vi "Functional Post Analysis.vi"(0 "Saving Path":path, 1 "Sensors":T2(array[cluster])=[{"Sensor Name"="", "Sensor Info"={"Manufacturer"="", "Model"="", "Serial Number"=""}, "Last Cal Info"={"Last Calibration Date"=0.0, "Calibrator"="", "Cal Duration"=0}, "Voltage Range"={"High Limit"=0.0, "Low Limit"=0.0}, "EGU Range"={"High Limit"=0.0, "Low Limit"=0.0}, "Units"="Volts", "Calibration Type"=enum."Calibrate Analog", "EGU List"=[], "Voltage List"=[], "Coefficients"=[], "Order"=0, "Algorithm"=enum."SVD", "Max Error % of Full Scale"=0.0, "Max Mean Squared Error"=0.0, "Use Error %"=FALSE, "Use MSE"=FALSE, "Allow Manual Entry"=FALSE, "Max Stability Error"=0.0, "Max Error % of Reading"=0.0, "Use Error % of Reading"=FALSE}], 2 "Config":T3={"DAQ Settings"={"Trigger Type"=enum."Manual", "Trigger Samples"=0, "Pretrigger Samples"=0, "Trigger Interval"=0.0, "Time Units"=FALSE, "Auto Save"=FALSE, "Sample Rate"=7.0, "Select Analog"=FALSE, "Trigger Value"=0.0, "Trigger Stop Method"=enum."Use Samples Value to Stop Trigger", "Rate Sec/Min"=FALSE, "Save Mode"=enum."Single File", "File Size Limit"=0.0, "Log File Type"=enum."Basic", "Trigger Data Index"=0}, "Channels"=[{"Channel"="", "Type"="", "Acquire"=FALSE, "Name"="", "Sensor"="", "Data Index"=0}, {"Channel"="", "Type"="", "Acquire"=FALSE, "Name"="", "Sensor"="", "Data Index"=0}, {"Channel"="", "Type"="", "Acquire"=FALSE, "Name"="", "Sensor"="", "Data Index"=0}, {"Channel"="", "Type"="", "Acquire"=FALSE, "Name"="", "Sensor"="", "Data Index"=0}], "Header"={"TA Number"="", "Test Name"="", "Serial Number"="", "Technician"=""}, "Graph Settings"={"Graph Labels"=[], [], [], [], [], [], [], [], [], [], [], [], [], "Graph Toggles"=[], "Axis Toggles"=[], "Graph Range"=enum."1"}, "Test Limits"=[{"Channel Acquired?"=TRUE, "RMS?"=FALSE, "Pk-Pk"=FALSE, "Frequency"=TRUE, "EU High Limit 1"=0.0, "EU Low Limit 1"=0.0, "EU High Limit 2"=0.0, "EU Low Limit 2"=0.0, "RMS High Limit"=0.0, "RMS Low Limit"=0.0, "Pk-Pk High Limit "=0.0, "Pk-Pk Low Limit"=0.0, "Frequency High Limit"=1.0, "Frequency Low Limit"=0.0}, {"Channel Acquired?"=TRUE, "RMS?"=FALSE, "Pk-Pk"=FALSE, "Frequency"=FALSE, "EU High Limit 1"=1.0, "EU Low Limit 1"=0.0, "EU High Limit 2"=0.0, "EU Low Limit 2"=0.0, "RMS High Limit"=0.0, "RMS Low Limit"=0.0, "Pk-Pk High Limit "=0.0, "Pk-Pk Low Limit"=0.0, "Frequency High Limit"=0.0, "Frequency Low Limit"=0.0}, {"Channel Acquired?"=TRUE, "RMS?"=FALSE, "Pk-Pk"=FALSE, "Frequency"=TRUE, "EU High Limit 1"=0.0, "EU Low Limit 1"=0.0, "EU High Limit 2"=0.0, "EU Low Limit 2"=0.0, "RMS High Limit"=0.0, "RMS Low Limit"=0.0, "Pk-Pk High Limit "=0.0, "Pk-Pk Low Limit"=0.0, "Frequency High Limit"=1.0, "Frequency Low Limit"=0.0}, {"Channel Acquired?"=TRUE, "RMS?"=FALSE, "Pk-Pk"=FALSE, "Frequency"=FALSE, "EU High Limit 1"=1.0, "EU Low Limit 1"=0.0, "EU High Limit 2"=0.0, "EU Low Limit 2"=0.0, "RMS High Limit"=0.0, "RMS Low Limit"=0.0, "Pk-Pk High Limit "=0.0, "Pk-Pk Low Limit"=0.0, "Frequency High Limit"=0.0, "Frequency Low Limit"=0.0}], "All Type Info"=[{"Type Name"="Type Name", "Type Signal Names"=["Signal 1", "Signal 2"], "# Signals"=2, "# Parts"=2, "Part Info"=[{"Part Number"="Part 1", "Channel Indexes"=[0, 1], "Enabled?"=TRUE}, {"Part Number"="Part 2", "Channel Indexes"=[2, 3], "Enabled?"=TRUE}]}], "Save Mode"=enum."Single File"} {"DAQ Settings"."Trigger Interval" min=0.0; "DAQ Settings"."Pretrigger Samples" min=0; "DAQ Settings"."Trigger Samples" min=0}, 3 "Frequency Coefficients":cluster{"Coefficients":dbl[]}[](array[cluster]), 7 "Functional Test Data":T1) -> (4 "Array":string[][](array[string]))   [LabVIEW 2019]
uses:
  <vilib>/Utility/file.llb/Read From Spreadsheet File (string).vi
  Type Defs and Controls/Trigger Stop Method.ctl
  Type Defs and Controls/DAQ Settings.ctl
  Type Defs and Controls/Header.ctl
  Type Defs and Controls/Channel Config.ctl
  Type Defs and Controls/Graph Settings Type Def.ctl
  Type Defs and Controls/Test Limits.ctl
  Type Defs and Controls/Sensor Config.ctl
  Type Defs and Controls/Part Info.ctl
  Type Defs and Controls/All Part Info.ctl
  Type Defs and Controls/Functional Info.ctl
  Type Defs and Controls/Log File Type.ctl
panel:
  out "number":sgl[][](array[numeric])
  out "error out":errorcluster
  # "EGU"
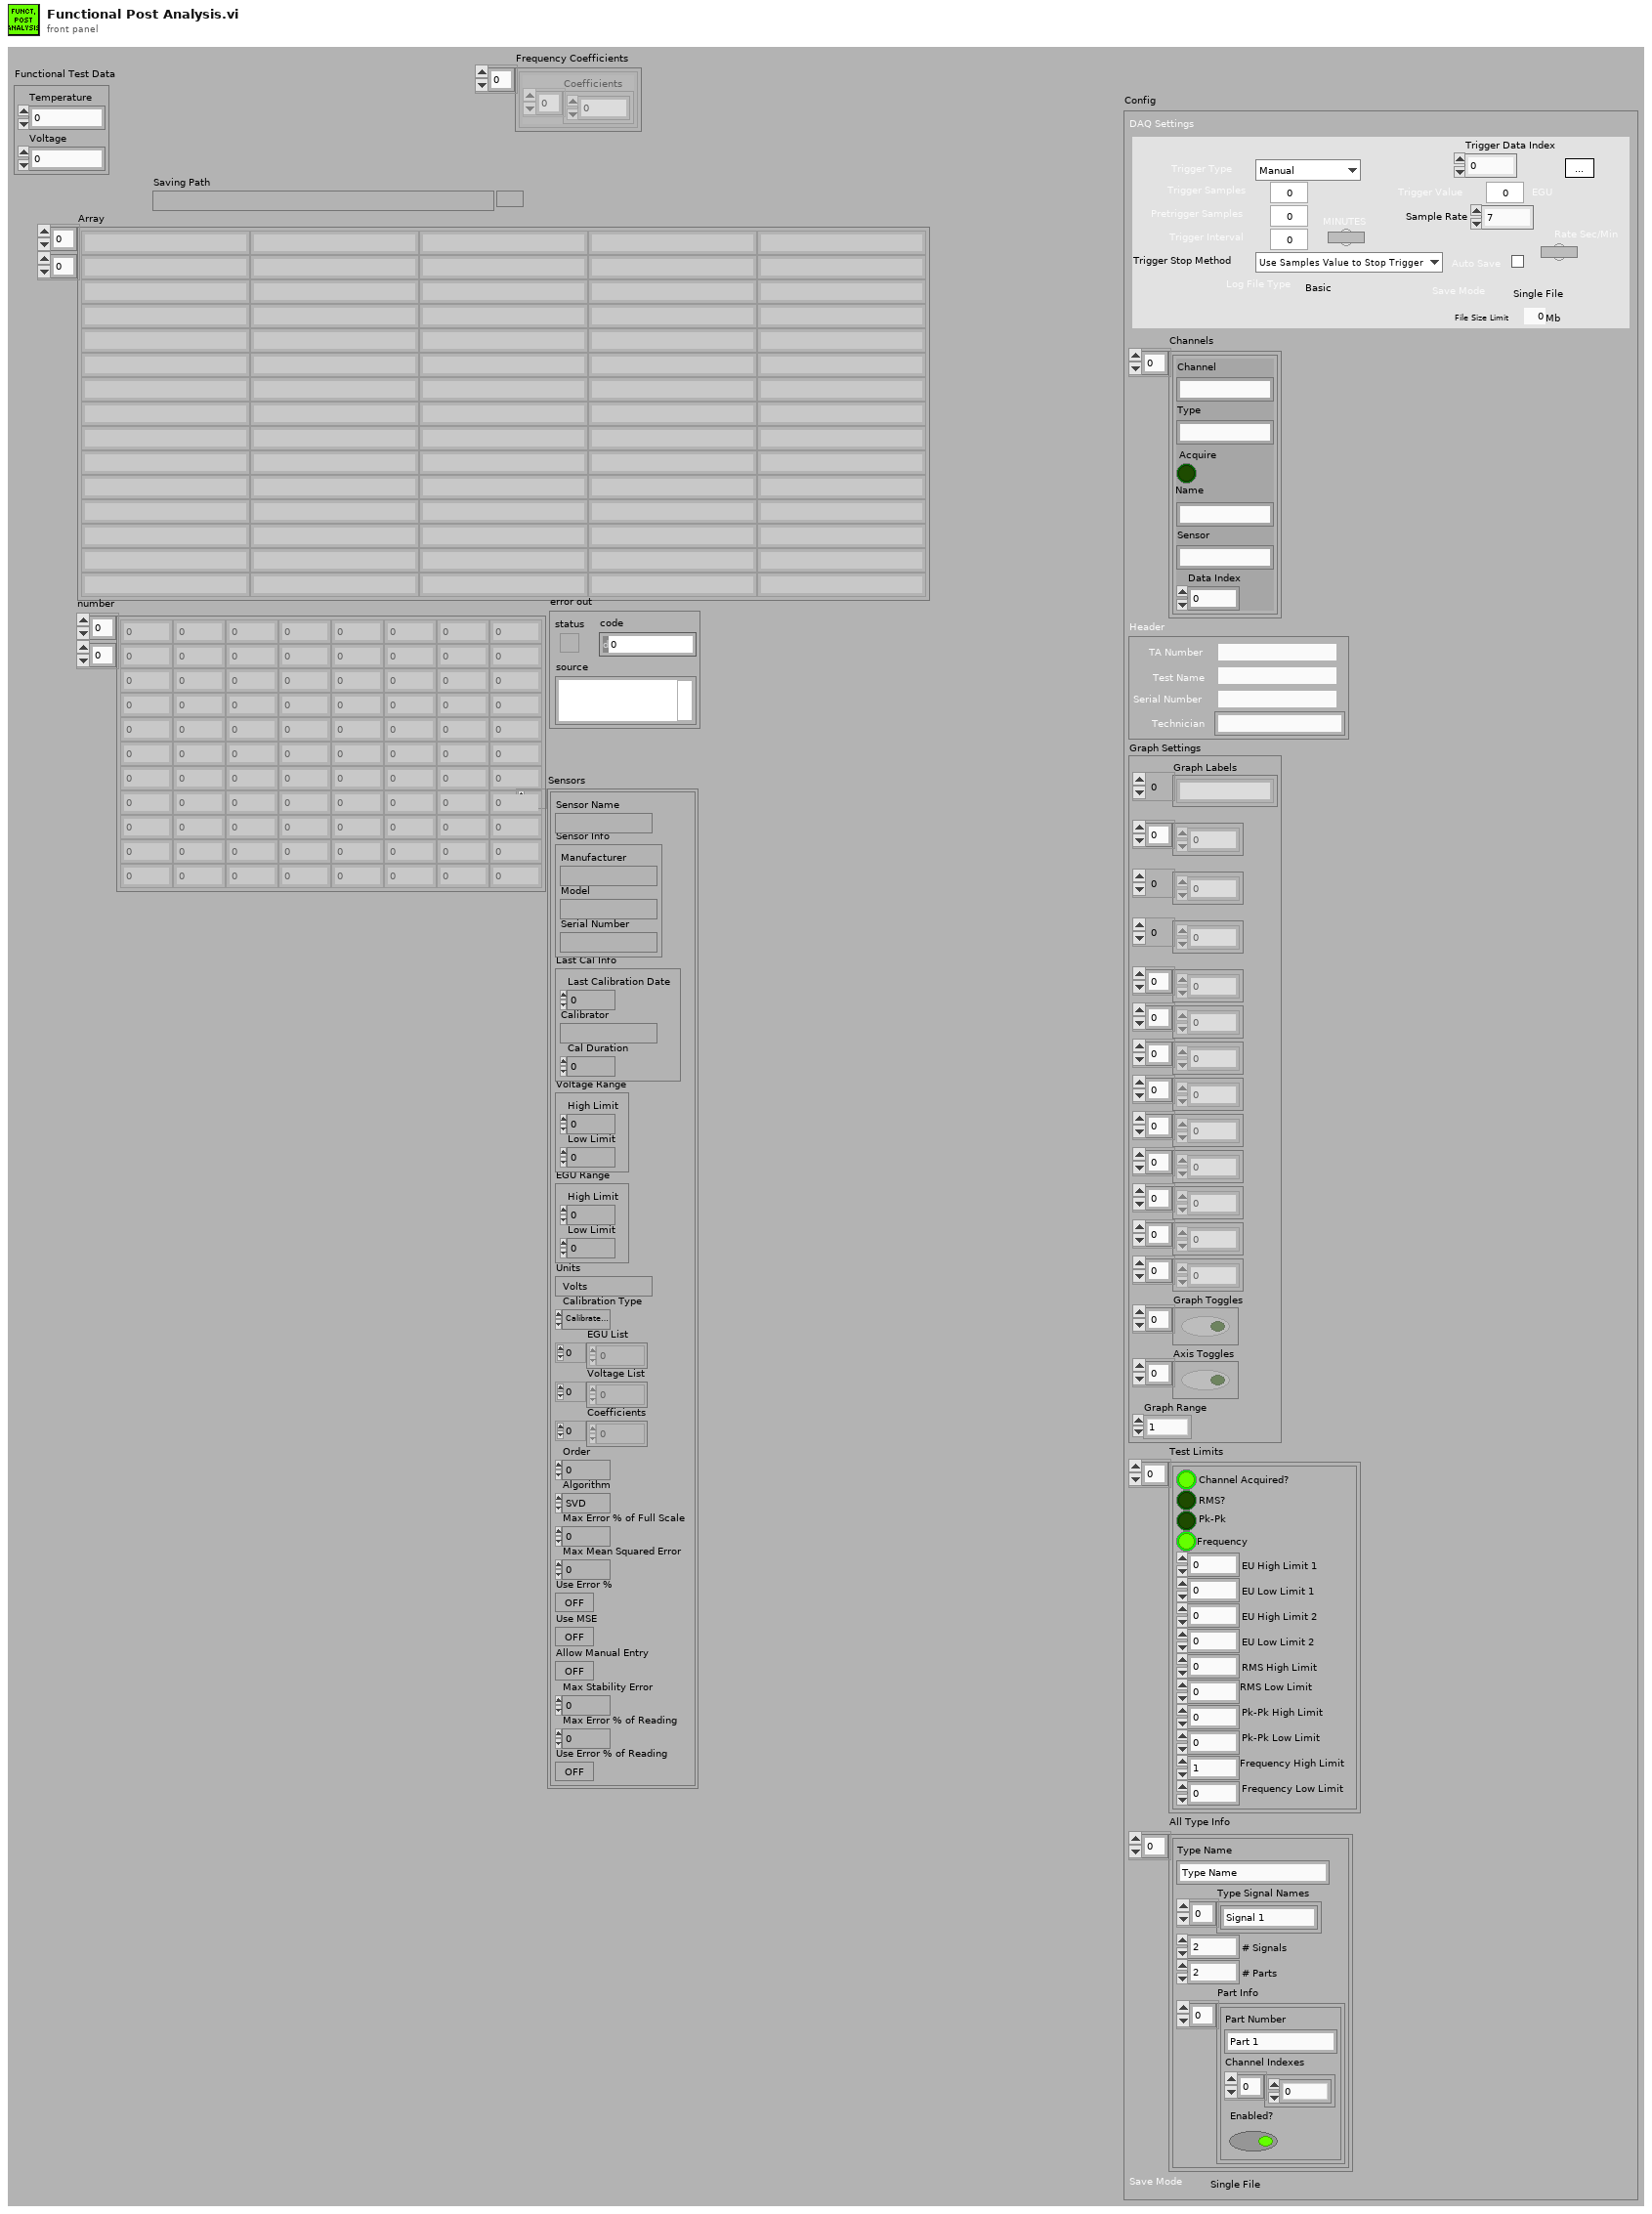
[diagram p1: front panel]
types:
  T1 = typedef "Functional Info.ctl" = cluster{"Temperature":dbl, "Voltage":dbl}
  T2 = cluster{"Sensor Name":string, "Sensor Info":cluster{"Manufacturer":string, "Model":string, "Serial Number":string}, "Last Cal Info":cluster{"Last Calibration Date":dbl, "Calibrator":string, "Cal Duration":i32}, "Voltage Range":cluster{"High Limit":dbl, "Low Limit":dbl}, "EGU Range":cluster{"High Limit":dbl, "Low Limit":dbl}, "Units":string, "Calibration Type":enum16{"Calibrate Analog", "Compare Analog Calibration"}, "EGU List":dbl[], "Voltage List":dbl[], "Coefficients":dbl[], "Order":i32, "Algorithm":enum32{"SVD", "Givens", "Givens2", "Householder", "LU Decomposition", "Cholesky"}, "Max Error % of Full Scale":dbl, "Max Mean Squared Error":dbl, "Use Error %":bool, "Use MSE":bool, "Allow Manual Entry":bool, "Max Stability Error":dbl, "Max Error % of Reading":dbl, "Use Error % of Reading":bool}[]
  T3 = typedef "Sensor Config.ctl" = cluster{"DAQ Settings":T4, "Channels":T7[], "Header":T8, "Graph Settings":T9, "Test Limits":T10[], "All Type Info":T11, "Save Mode":enum16{"Single File", "Segmented Files", "New File at Midnight"}}
  T4 = typedef "DAQ Settings.ctl" = cluster{"Trigger Type":enum16{"Manual", "Timed", "Analog Rising", "Analog Falling"}, "Trigger Samples":i32, "Pretrigger Samples":i32, "Trigger Interval":dbl, "Time Units":bool, "Auto Save":bool, "Sample Rate":dbl, "Select Analog":bool, "Trigger Value":dbl, "Trigger Stop Method":T5, "Rate Sec/Min":bool, "Save Mode":enum16{"Single File", "Segmented Files", "New File at Midnight"}, "File Size Limit":dbl, "Log File Type":T6, "Trigger Data Index":u32}
  T5 = typedef "Trigger Stop Method.ctl" = enum16{"Use Samples Value to Stop Trigger", "Use Threshold to Stop Trigger"}
  T6 = typedef "Log File Type.ctl" = enum16{"Basic", "RTS"}
  T7 = typedef "Channel Config.ctl" = cluster{"Channel":string, "Type":string, "Acquire":bool, "Name":string, "Sensor":string, "Data Index":u32}
  T8 = typedef "Header.ctl" = cluster{"TA Number":string, "Test Name":string, "Serial Number":string, "Technician":string}
  T9 = typedef "Graph Settings Type Def.ctl" = cluster{"Graph Labels":string[], u8[], i16[], u32[], u8[], u8[], u8[], u32[], u8[], u8[], u8[], dbl[], dbl[], "Graph Toggles":bool[], "Axis Toggles":bool[], "Graph Range":enum16{"1", "2", "3", "4", "5", "10", "15", "30", "60"}}
  T10 = typedef "Test Limits.ctl" = cluster{"Channel Acquired?":bool, "RMS?":bool, "Pk-Pk":bool, "Frequency":bool, "EU High Limit 1":dbl, "EU Low Limit 1":dbl, "EU High Limit 2":dbl, "EU Low Limit 2":dbl, "RMS High Limit":dbl, "RMS Low Limit":dbl, "Pk-Pk High Limit ":dbl, "Pk-Pk Low Limit":dbl, "Frequency High Limit":dbl, "Frequency Low Limit":dbl}
  T11 = typedef "All Part Info.ctl" = cluster{"Type Name":string, "Type Signal Names":string[], "# Signals":i32, "# Parts":i32, "Part Info":T12[]}[]
  T12 = typedef "Part Info.ctl" = cluster{"Part Number":string, "Channel Indexes":u16[], "Enabled?":bool}
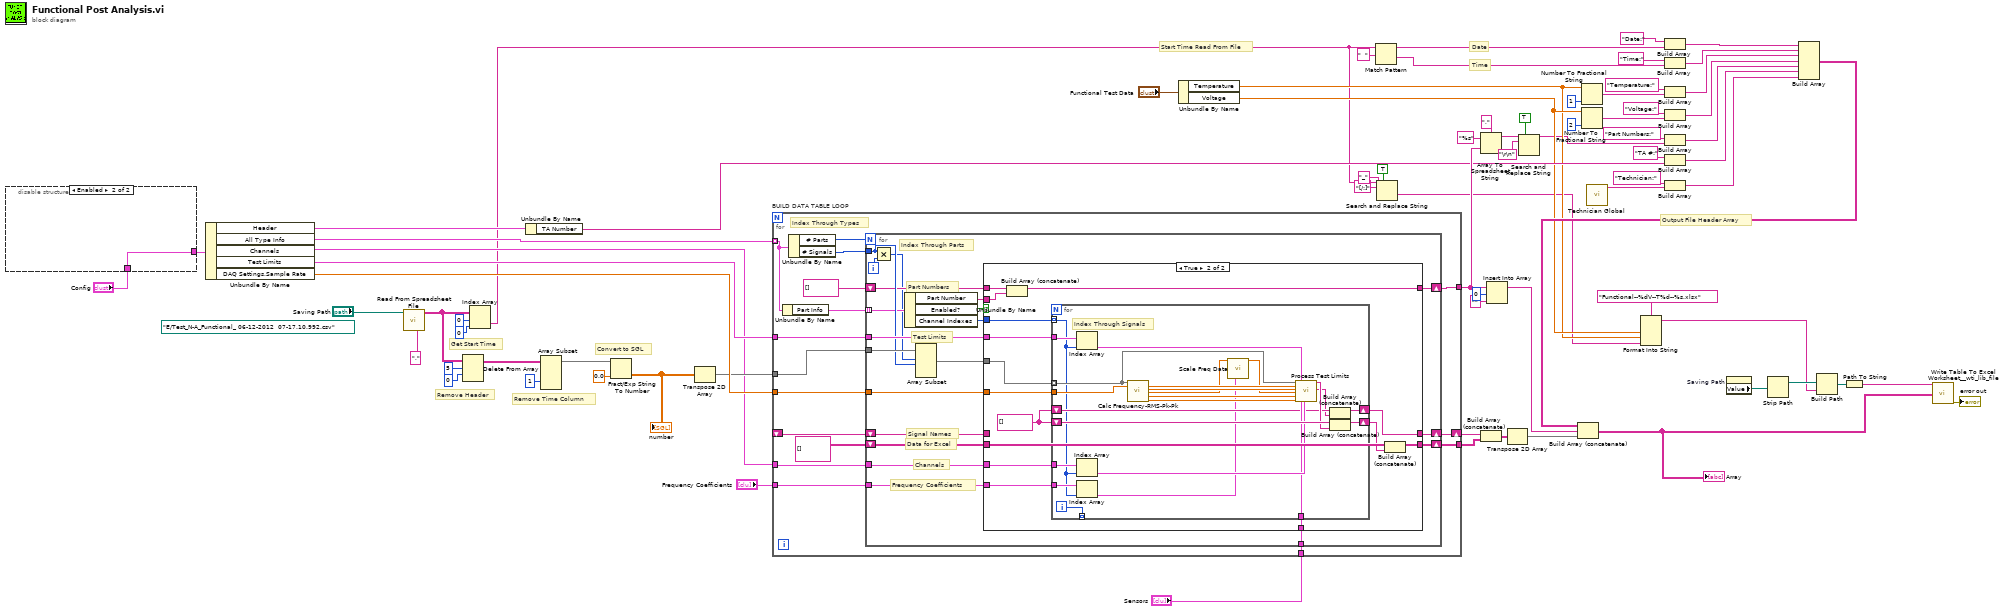
[diagram p0: block diagram]
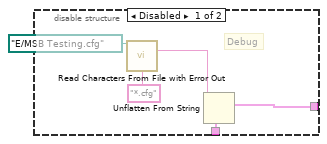
[diagram p2: hidden frame]
diagram:
  (unwired) path "E:/Test_N-A_Functional_ 06-12-2012  07-17.10.992.csv" ("file path (dialog if empty)")
  # "Start Time Read From File"
  # "Time"
  # "Date"
  # "Output File Header Array"
  # "Get Start Time"
  # "Remove Header"
  # "Convert to SGL"
  # "Remove Time Column"
  n1 = disable-structure shown="Enabled" {
    disable-tunnel: "Config" -> [w79 w82]
    disable-tunnel: [w78 w82] -> w2
    frame Disabled {
      # "Debug"
      n2 = call "Read Characters From File with Error Out.vi"("file path (dialog if empty)"=path "E:/MSB Testing.cfg", "[pattern]"="*.cfg") -> ("character string"=w80:string)  [unwired: 9 in, 4 out]
      n3 = Unflatten From String(type=w79, binary string=w80) -> (value=w78:T3)  [unwired: 3 in, 2 out]
    }
    frame Enabled {
    }
  }
  n4 = Unbundle By Name(w2) -> ("Header"=w57:T8, "All Type Info"=w68:T11, "Channels"=w66:T7[], "Test Limits"=w67:T10[], "DAQ Settings.Sample Rate"=w70:dbl)
  n5 = call-poly <vilib>:"Read From Spreadsheet File.vi"("delimiter (\\t)"="," ("delimiter (\\t)"), "file path (dialog if empty)"="Saving Path") -> ("all rows"=w73:string[][])  [unwired: 5 in, 4 out]
  n6 = Delete From Array(array=w73, length=5 ("index (row)"), index (row)=0) -> (array with subset deleted=w9:string[][])  [unwired: 1 in, 1 out]
  n7 = Index Array(array=w73, index (row)=0, index (col)=0 ("disabled index (col)")) -> (element=w21:string)
  n8 = Unbundle By Name(w57) -> ("TA Number"=w30:string)
  n9 = Array Subset(array=w9, index (col)=1 ("index")) -> (w8:string[][])  [unwired: 3 in]
  n10 = Fract/Exp String To Number(string=w8, default (0 dbl)=sgl 0.0 ("default (0 DBL)")) -> (number=w6:sgl[][])  [unwired: 2 in, 1 out]
  "number" <- w6
  n11 = Transpose 2D Array(2D array=w6) -> (transposed array=w69:sgl[][])
  n12 = for "BUILD DATA TABLE LOOP" {
    tunnel: w67 -> [w98]
    tunnel: w70 -> [w97]
    tunnel: w69 -> [w96]
    tunnel: w68 -> [w92] mode=indexing
    tunnel: [w93] -> w63
    tunnel: w66 -> [w90]
    tunnel: "Sensors" -> [w89]
    tunnel: [w86] -> w40
    shift-right: [w88] -> w61
    shift-left: _ -> [w85]
    tunnel: "Frequency Coefficients" -> [w84]
    # "Index Through Types"
    n13 = Unbundle By Name(w92) -> ("Part Info"=w91:T12[])
    n14 = Unbundle By Name(w92) -> ("# Parts"=w83:i32, "# Signals"=w95:i32)
    n15 = for {
      N: w83 -> [_]
      tunnel: w98 -> [w117]
      tunnel: w96 -> [w116]
      tunnel: w97 -> [w118]
      tunnel: w95 -> [w114]
      shift-right: [w111] -> w93
      shift-left: string[][] [] -> [w112]
      tunnel: w91 -> [w110] mode=indexing
      tunnel: w90 -> [w108]
      tunnel: w89 -> [w107]
      shift-right: [w102] -> w86
      shift-left: string[] [] -> [w104]
      shift-right: [w106] -> w88
      shift-left: w85 -> [w101]
      tunnel: w84 -> [w99]
      i -> [w115]
      # "Part Numbers"
      # "Test Limits"
      # "Signal Names"
      # "Data for Excel"
      # "Channels"
      # "Frequency Coefficients"
      # "Index Through Parts"
      n16 = Multiply(x=w114, y=w115) -> (x*y=w100:i32)
      n17 = Unbundle By Name(w110) -> ("Part Number"=w103:string, "Enabled?"=w105:bool, "Channel Indexes"=w109:u16[])
      n18 = Array Subset(array=w116, index (row)=w100, length (row)=w114) -> (w113:sgl[][])  [unwired: 2 in]
      n19 = case shown="True" w105 {
        tunnel: w118 -> [_ w136]
        tunnel: w117 -> [_ w135]
        tunnel: w113 -> [_ w134]
        tunnel: w112 -> [w119 w133]
        tunnel: [w119 w131] -> w111
        tunnel: w109 -> [_ w130]
        tunnel: w108 -> [_ w129]
        tunnel: w107 -> [_ w128]
        tunnel: [w120 w126] -> w106
        tunnel: w104 -> [w121 w125]
        tunnel: w103 -> [_ w124]
        tunnel: [w121 w123] -> w102
        tunnel: w101 -> [w120 _]
        tunnel: w99 -> [_ w122]
        frame False {
        }
        frame True {
          w127 = string[] []
          n20 = Build Array (concatenate)(w125, w124) -> (w123:string[])
          n21 = for {
            tunnel: w136 -> [w159]
            tunnel: w135 -> [w150]
            tunnel: w134 -> [w154] mode=indexing
            shift-right: [w153] -> w132
            shift-left: w127 -> [w152]
            tunnel: w130 -> [w141] mode=indexing
            tunnel: w129 -> [w148]
            tunnel: w128 -> [w146]
            shift-right: [w145] -> w126
            shift-left: w127 -> [w144]
            tunnel: w122 -> [w142]
            tunnel: [w137] -> _ mode=indexing
            i -> [w137]
            # "Index Through Signals"
            n22 = Index Array(array=w150, index=w141) -> (element=w149:T10)
            n23 = Index Array(array=w148, index=w141) -> (element=w147:T7)
            n24 = Index Array(array=w142, index=w141) -> (element=w140:cluster{"Coefficients":dbl[]})
            n25 = call "Calc Frequency-RMS-Pk-Pk.vi"("Signal Data In"=w154, "Sample Rate"=w159) -> ("RMS"=w158:dbl[], "Pk-Pk"=w157:dbl[], "Frequency"=w139:dbl[], "Peak"=w156:dbl[], "Valley"=w155:dbl[])  [unwired: 13 in]
            n26 = call "Scale Freq Data.vi"("Data Read"=w139, "Signal Coefficients"=w140) -> ("Scaled Data"=w138:dbl[])  [unwired: 13 in]
            n27 = call "Process Test Limits.vi"("Signal In"=w154, "RMS"=w158, "Pk-Pk"=w157, "Frequency"=w138, "Peaks"=w156, "Valleys"=w155, "Test Limits"=w149, "Sensors"=w146, "Channel"=w147) -> ("Data Array"=w151:string[], "Channel Labels"=w143:string[])  [unwired: 9 in]
            n28 = Build Array (concatenate)(w144, w143) -> (w145:string[])
            n29 = Build Array (concatenate)(w152, w151) -> (w153:string[])
          }
          n30 = Build Array (concatenate)(w133, w132) -> (w131:string[][])
        }
      }
    }
  }
  n31 = Unbundle By Name("Functional Test Data") -> ("Temperature"=w25:dbl, "Voltage"=w26:dbl)
  n32 = Match Pattern(string=w21, regular expression="  ") -> (before substring=w54:string, after substring=w52:string)  [unwired: 1 in, 2 out]
  n33 = Search and Replace String(replace all?=TRUE ("replace all? (F)"), input string=w21, search string="[/:]", replace string="_" ("replace string (\"\")")) -> (result string=w22:string)  [unwired: 4 in, 3 out]
  n34 = Array To Spreadsheet String(delimiter (Tab)=",", array=w40, 3:"%s" ("format string")) -> (spreadsheet string=w14:string)
  n35 = Build Array (concatenate)(w61, w63) -> (w64:string[][])
  n36 = Insert Into Array(array=w40, index=0, new element="" ("new element/subarray")) -> (w58:string[])
  n37 = Transpose 2D Array(2D array=w64) -> (transposed array=w62:string[][])
  n38 = Search and Replace String(replace all?=TRUE ("replace all? (F)"), input string=w14, search string="\r\n") -> (result string=w12:string)  [unwired: 5 in, 3 out]
  n39 = Number To Fractional String(number=w25, precision (6)=i16 1) -> (F-format string=w46:string)  [unwired: 2 in]
  n40 = Number To Fractional String(number=w26, precision (6)=i16 2) -> (F-format string=w43:string)  [unwired: 2 in]
  n41 = call "Technician Global.vi"() -> ("Technician Name"=w35:string)  [unwired: 11 in]
  n42 = Format Into String(format string="Functional--%dV--T%d--%s.xlsx", w26, w25, w22) -> (resulting string=w23:string)  [unwired: 2 in, 1 out]
  n43 = Build Array("Date:" ("element"), w54) -> (w51:string[])
  n44 = Build Array("Time:" ("element"), w52) -> (w50:string[])
  n45 = Build Array("Temperature:" ("element"), w46) -> (w42:string[])
  n46 = Build Array("Voltage:" ("element"), w43) -> (w41:string[])
  n47 = Build Array("Part Numbers:" ("element"), w12) -> (w36:string[])
  n48 = Build Array("TA #:" ("element"), w30) -> (w29:string[])
  n49 = Build Array("Technician:" ("element"), w35) -> (w32:string[])
  n50 = property on="Saving Path" class="Path"() -> ("Value"=w28:path)  [unwired: 2 in, 2 out]
  n51 = Strip Path(path=w28) -> (stripped path=w24:path)  [unwired: 1 out]
  n52 = Build Array(w51, w50, w42, w41, w36, w29, w32) -> (w33:string[][])
  n53 = Build Array (concatenate)(w33, w58, w62) -> (w11:string[][])
  "Array" <- w11
  n54 = Build Path(base path=w24, name or relative path=w23) -> (appended path=w16:path)
  n55 = Path To String(path=w16) -> (string=w17:string)
  n56 = call <vilib>:"Write Table To Excel Worksheet__wti_lib_file.vi"("Filename"=w17, "Table Data"=w11) -> ("error out"=→"error out":errorcluster)  [unwired: 17 in]
